vi "Periodic Tasks.vi"(11 "error out":errorcluster) -> ()   [LabVIEW 2013]
doc: "This VI runs in parallel to other tasks. It can contain as many user-defined periodic loops as you need. These can carry out PID or other sorts of timed response."
uses:
  <vilib>/Rock Robotics/SystemInterfaces/Utilities/FPGA_UtilitiesLED Source.ctl
  <vilib>/Rock Robotics/SystemInterfaces/Utilities/FPGA_UtilitiesLED State.ctl
  Robot Global Data.vi
  <vilib>/Rock Robotics/WPI/Joystick/WPI_JoystickGetSetRefNum.vi
  <vilib>/addons/control/pid/pid.llb/PID (DBL).vi
  <vilib>/addons/control/pid/NI_PID_pid.lvlib
  <vilib>/addons/Kinect/Skeleton Vertex Index.ctl
  <vilib>/addons/Kinect/SkeletonVertexTrackState.ctl
panel:
  out "x < y?":bool
  in  "Angle 2":i32=170
  in  "y 6":dbl=53.0
  in  "y 5":dbl=54.0
  in  "Drive PID":T1={"proportional gain (Kc)"=1.0, "integral time (Ti, min)"=0.01, "derivative time (Td, min)"=0.0} {"derivative time (Td, min)" format="%.3f"; "integral time (Ti, min)" format="%.3f"; "proportional gain (Kc)" format="%.3f"}
  in  "Joystick Multiplier":dbl=24.0
  in  "RateDivision":dbl=128.0
  out "Angle":dbl
  in  "Gyro PID":bool
  in  "PID gains 4":T1={"proportional gain (Kc)"=0.09999999999999999, "integral time (Ti, min)"=0.0, "derivative time (Td, min)"=0.002} {"derivative time (Td, min)" format="%.3f"; "integral time (Ti, min)" format="%.3f"; "proportional gain (Kc)" format="%.3f"}
  in  "SetFeeder":dbl=0.5
  in  "Encoder PID":bool
  in  "Reset Encoders":bool
  in  "y 4":i32=40
  in  "lower limit":dbl
  in  "y 3":i32=30
  in  "x":dbl=1.0
  in  "y 2":i32=2
  in  "y":i32=10
  in  "Gain (VoltsPerDegree/Second)":dbl=0.006999999999999999
  in  "Reset Gyro":bool
  in  "Encoder PID gains 2":T1={"proportional gain (Kc)"=0.30000000000000004, "integral time (Ti, min)"=0.0, "derivative time (Td, min)"=0.0}
  in  "Fly Speed 1":dbl(slide)=64.0 scale=0.0..100.0
  in  "Fly Speed 2":dbl(slide)=63.0 scale=0.0..100.0
  in  "Shooter Speed":T1={"proportional gain (Kc)"=0.13999999999999999, "integral time (Ti, min)"=0.0, "derivative time (Td, min)"=0.0} {"derivative time (Td, min)" format="%.3f"; "integral time (Ti, min)" format="%.3f"; "proportional gain (Kc)" format="%.3f"}
  in  "Fly 1":dbl
  in  "Fly 2":dbl
  out "Fly1 Rate":dbl
  out "Fly2 Rate":dbl
  in  "Reset Fly 2":bool
  in  "Reset Fly 1":bool
  out "Fly1":dbl
  out "Fly2":dbl
  in  "Encoder PID gains":T1={"proportional gain (Kc)"=0.30000000000000004, "integral time (Ti, min)"=0.0, "derivative time (Td, min)"=0.0}
  out "Drive Right feet":dbl
  out "Drive Left feet":dbl
  out "Drive Right":dbl
  out "Drive Left":dbl
  in  "PID gains 3":T1={"proportional gain (Kc)"=0.15, "integral time (Ti, min)"=0.0, "derivative time (Td, min)"=0.001} {"derivative time (Td, min)" format="%.3f"; "integral time (Ti, min)" format="%.3f"; "proportional gain (Kc)" format="%.3f"}
  # ".7 Front\n.5 Back"
  # "54/53 Front\n64/63 Back"
  # "-.72"
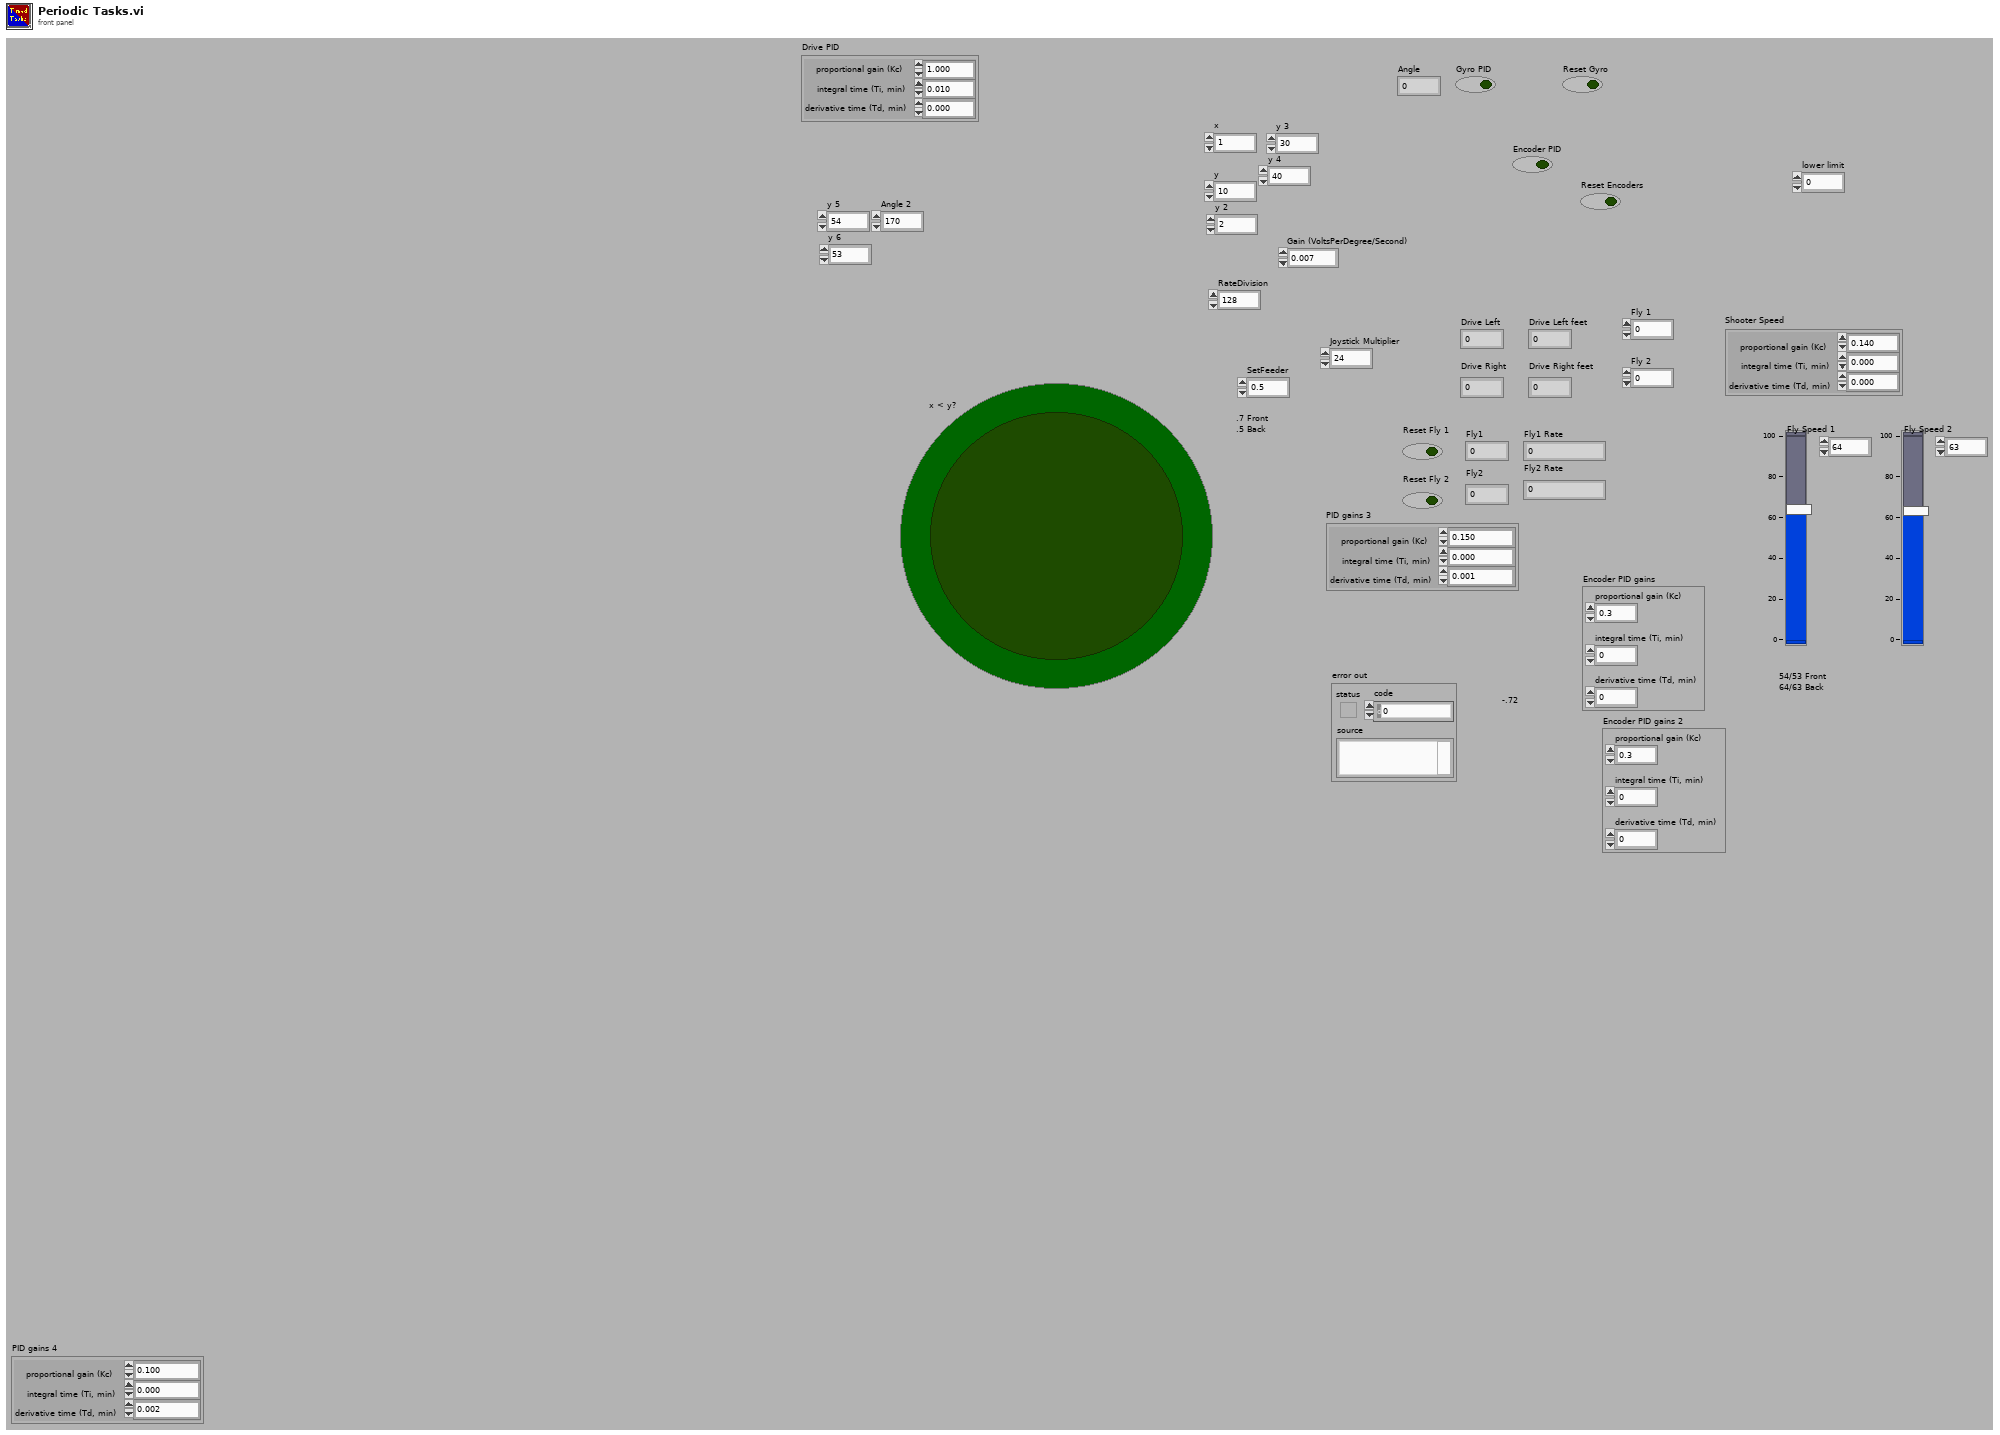
[diagram p1: front panel]
types:
  T1 = cluster{"proportional gain (Kc)":dbl, "integral time (Ti, min)":dbl, "derivative time (Td, min)":dbl}
  T2 = typedef "FPGA_UtilitiesLED State.ctl" = enum16{"Off", "On", "Toggle"}
  T3 = typedef "FPGA_UtilitiesLED Source.ctl" = enum16{"User LED", "FPGA LED"}
  T4 = typedef "WPI_MotorControlDeviceRef.ctl" = cluster{"DeviceStatus":errorcluster, "Type":enum16{"PWM", "CAN"}, "PWM":cluster{"Digital Module":T5, "PWM Channel":T6, "DeadBand":T7}, "CAN":cluster{"Device Number":u8, "Control Mode":T8, "Semaphore":T9, "Max Vout":dbl}, "Invert":bool, "TransformRef":T10, "InvTransformRef":T10}
  T5 = typedef "FPGA_TypedefDigitalModule.ctl" = enum16{"Digital Module 1", "Digital Module 2"}
  T6 = typedef "FPGA_DIOPWMChannel.ctl" = enum8{"PWM 1", "PWM 2", "PWM 3", "PWM 4", "PWM 5", "PWM 6", "PWM 7", "PWM 8", "PWM 9", "PWM 10", "Invalid"}
  T7 = typedef "WPI_PWMDeadband.ctl" = cluster{"Name":string, "maxPositivePwm":i32, "minPositivePwm":i32, "centerPwm":i32, "maxNegativePwm":i32, "minNegativePwm":i32, "angularRange":u16}
  T8 = typedef "WPI_CANJaguar_ControlMode.ctl" = enum8{"Percent VBus", "Current", "Speed", "Position", "Voltage"}
  T9 = typedef "Semaphore RefNum" = refnum<k1>
  T10 = typedef "WPI_PWMTransform_ConPane.ctl" = refnum<vi>
  T11 = typedef "WPI_EncoderDevRef.ctl" = cluster{"DevStatus":errorcluster, "EncoderIndex":T12, "CounterIndex":T13, "DistancePerCount":dbl, "Decoding Type":T14}
  T12 = typedef "FPGA_EncoderIdx.ctl" = enum8{"Enc 0", "Enc 1", "Enc 2", "Enc 3", "Invalid"}
  T13 = typedef "FPGA_CounterCtrSystemIndex.ctl" = enum8{"Ctr 0", "Ctr 1", "Ctr 2", "Ctr 3", "Ctr 4", "Ctr 5", "Ctr 6", "Ctr 7", "Invalid"}
  T14 = typedef "WPI_EncoderType.ctl" = enum16{"1x", "2x", "4x"}
  T15 = typedef "WPI_ServoDeviceRef.ctl" = cluster{"DeviceStatus":errorcluster, "Digital Module":T5, "PWM Channel":T6, "DeadBand":T7}
  T16 = typedef "WPI_JoystickDevRef.ctl" = cluster{"Device":T17}
  T17 = typedef "WPI_JoystickDeviceEnum.ctl" = enum16{"USB 1", "USB 2", "USB 3", "USB 4", "Kinect 1", "Kinect 2"}
  T18 = typedef "WPI_GyroDevRef.ctl" = cluster{"DevStatus":errorcluster, "Analog Module":T19, "Analog Channel":T20, "Offset":dbl, "Gain (VoltsPerDegree/Second)":dbl}
  T19 = typedef "FPGA_TypedefAnalogModule.ctl" = enum16{"Analog Module 1", "Analog Module 2"}
  T20 = typedef "FPGA_AIChannel.ctl" = enum8{"AI 1", "AI 2", "AI 3", "AI 4", "AI 5", "AI 6", "AI 7", "AI 8", "Invalid"}
  T21 = cluster{"axis 1 (x)":dbl, "axis 2 (y)":dbl, "axis 3 (throttle)":dbl, "axis 4":dbl, "axis 5":dbl, "axis 6":dbl}
  T22 = typedef "Skeleton Vertex Index.ctl" = i32
  T23 = typedef "SkeletonVertexTrackState.ctl" = enum32{"NotTracked", "Inferred", "Tracked"}
  T24 = cluster{"Target Info 2":cluster{"Center Position":cluster{"X":dbl, "Y":dbl}, "Distance (ft)":dbl, "Center":bool, "Angle":dbl}[]}
  T25 = cluster{"Center Position":cluster{"X":dbl, "Y":dbl}, "Distance (ft)":dbl, "Center":bool, "Angle":dbl}[]
  T26 = typedef "WPI_JoystickButtonState.ctl" = cluster{"Button 1":bool, "Button 2":bool, "Button 3":bool, "Button 4":bool, "Button 5":bool, "Button 6":bool, "Button 7":bool, "Button 8":bool, "Button 9":bool, "Button 10":bool, "Button 11":bool, "Button 12":bool}
  T27 = cluster{"Target Info 2[0]":cluster{"Center Position":cluster{"X":dbl, "Y":dbl}, "Distance (ft)":dbl, "Center":bool, "Angle":dbl}, "Target Info 2[1]":cluster{"Center Position":cluster{"X":dbl, "Y":dbl}, "Distance (ft)":dbl, "Center":bool, "Angle":dbl}, "Target Info 2[2]":cluster{"Center Position":cluster{"X":dbl, "Y":dbl}, "Distance (ft)":dbl, "Center":bool, "Angle":dbl}, "Target Info 2[3]":cluster{"Center Position":cluster{"X":dbl, "Y":dbl}, "Distance (ft)":dbl, "Center":bool, "Angle":dbl}, "Target Info 2[4]":cluster{"Center Position":cluster{"X":dbl, "Y":dbl}, "Distance (ft)":dbl, "Center":bool, "Angle":dbl}, "Target Info 2[5]":cluster{"Center Position":cluster{"X":dbl, "Y":dbl}, "Distance (ft)":dbl, "Center":bool, "Angle":dbl}, "Target Info 2[6]":cluster{"Center Position":cluster{"X":dbl, "Y":dbl}, "Distance (ft)":dbl, "Center":bool, "Angle":dbl}, "Target Info 2[7]":cluster{"Center Position":cluster{"X":dbl, "Y":dbl}, "Distance (ft)":dbl, "Center":bool, "Angle":dbl}, "Target Info 2[8]":cluster{"Center Position":cluster{"X":dbl, "Y":dbl}, "Distance (ft)":dbl, "Center":bool, "Angle":dbl}}
  T28 = cluster{"Center Position":cluster{"X":dbl, "Y":dbl}, "Distance (ft)":dbl, "Center":bool, "Angle":dbl}
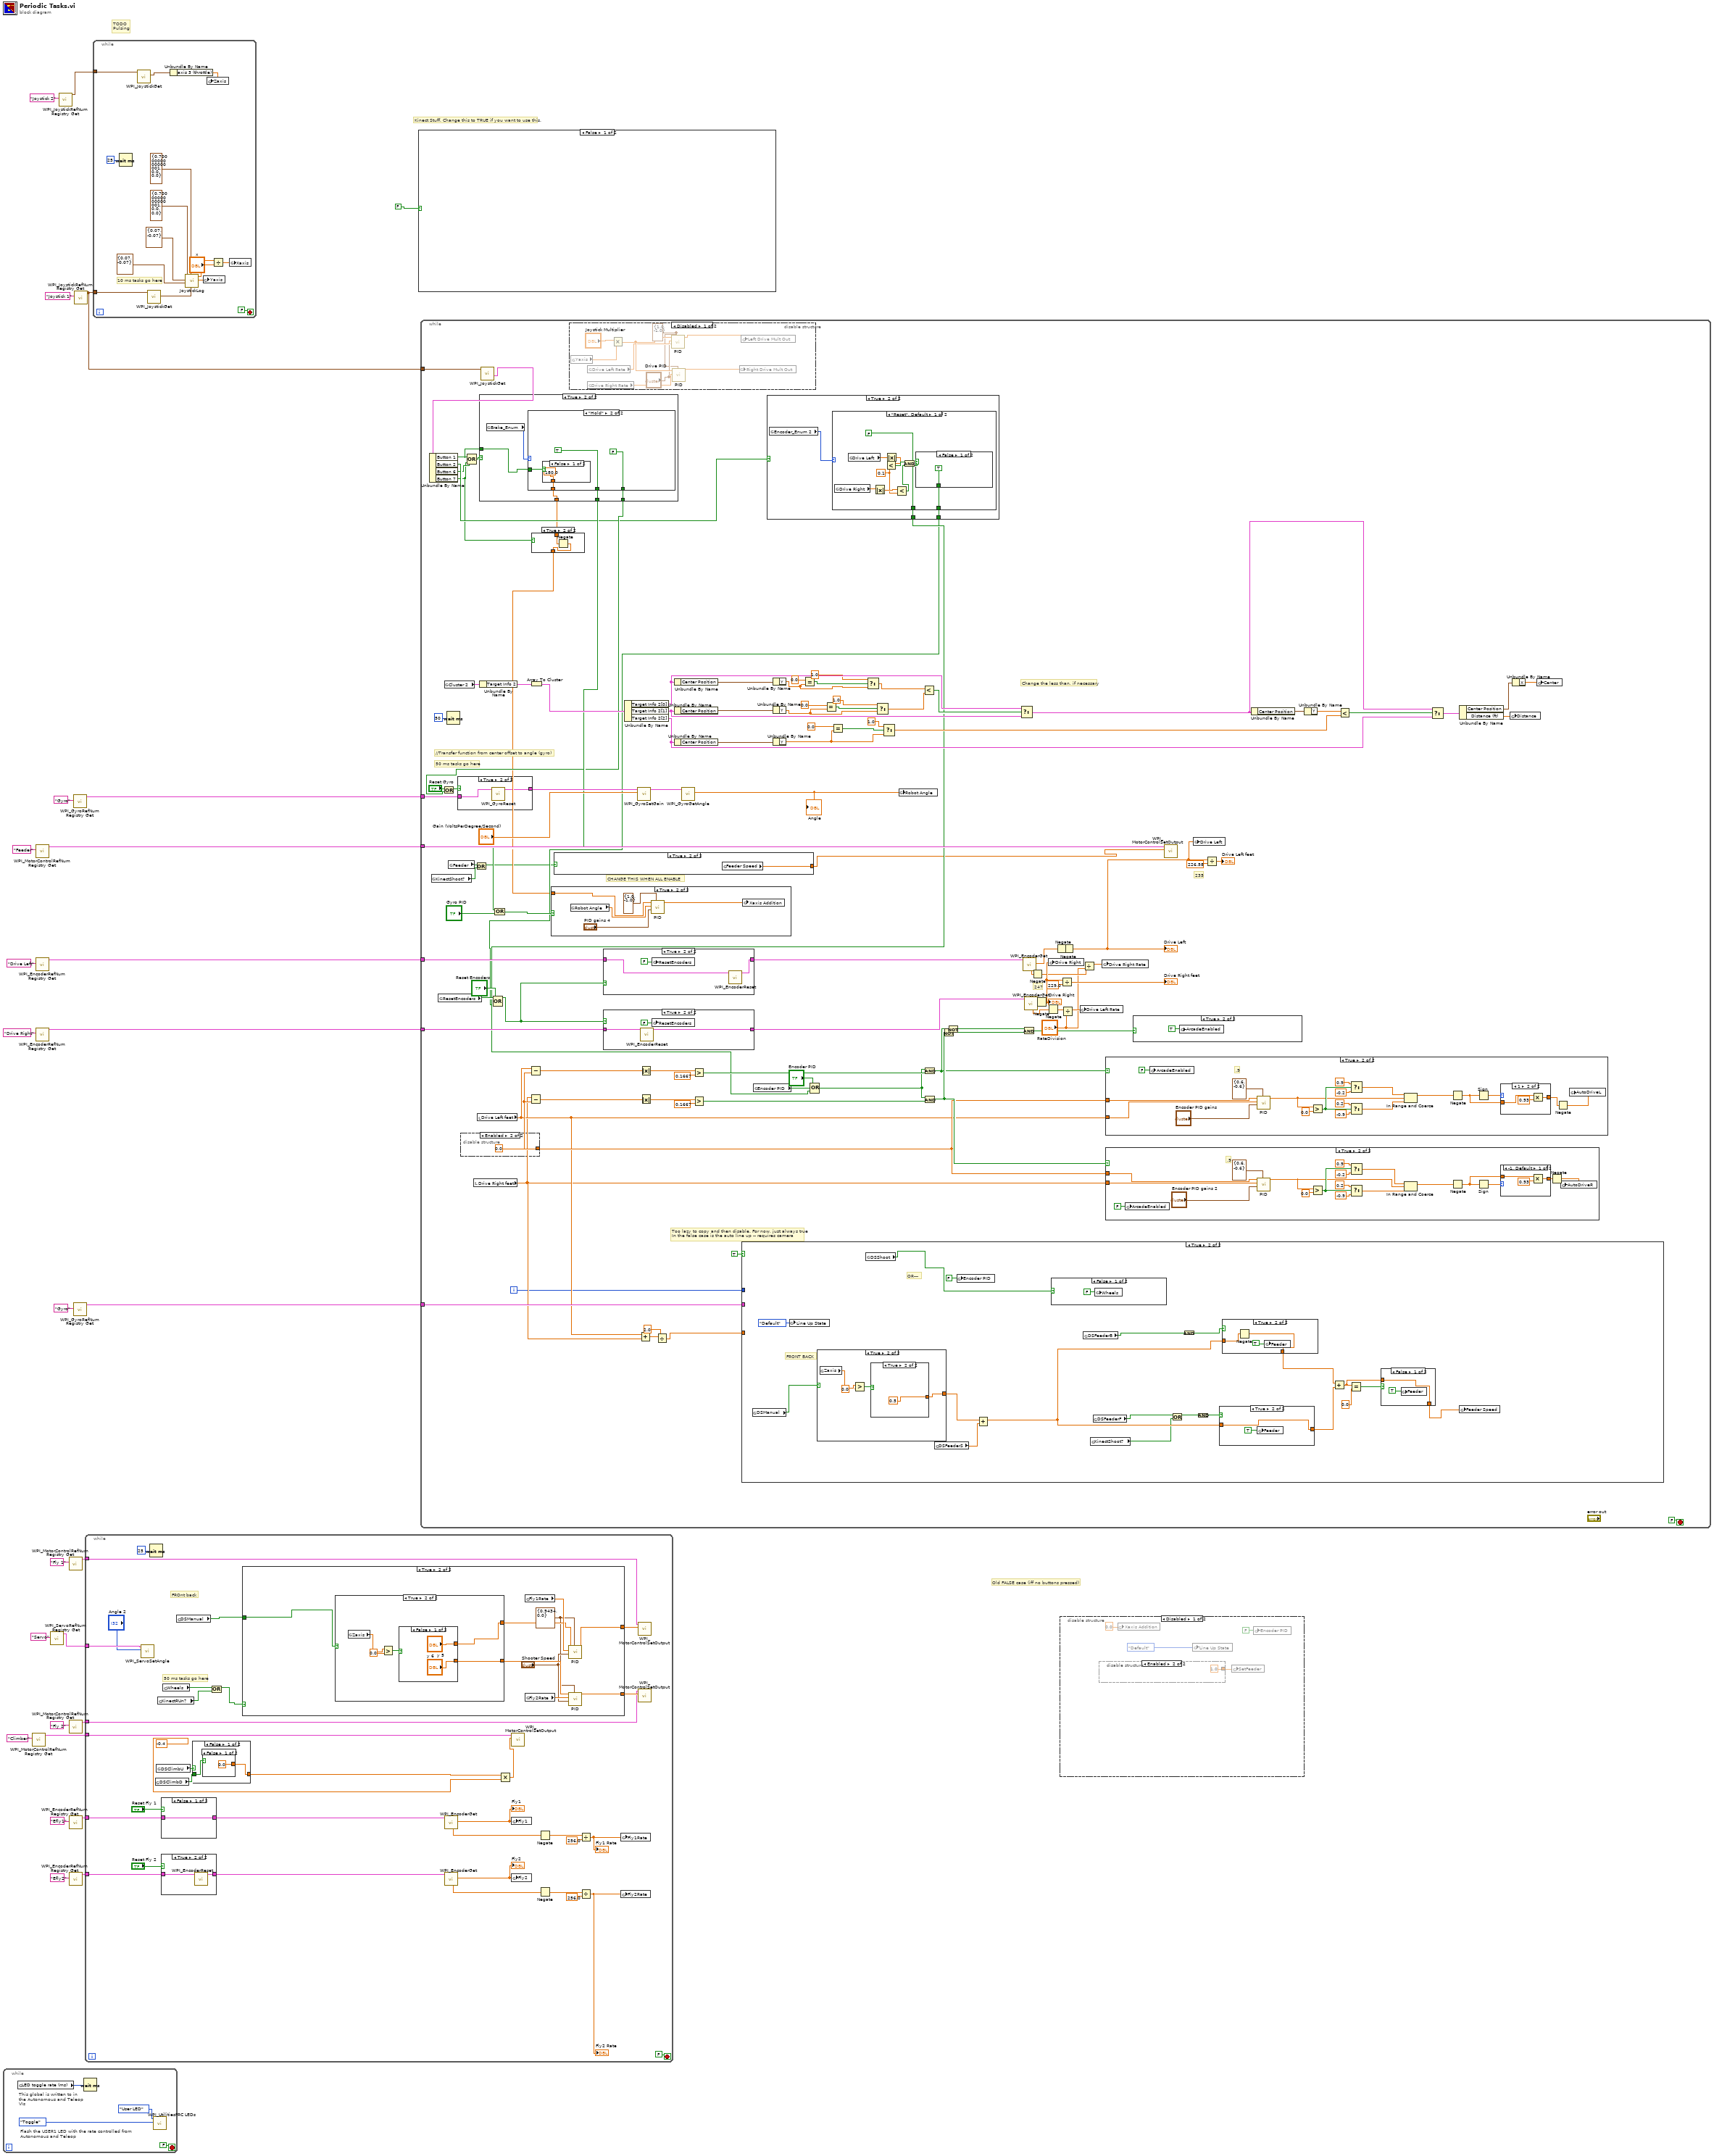
[diagram p0: block diagram]
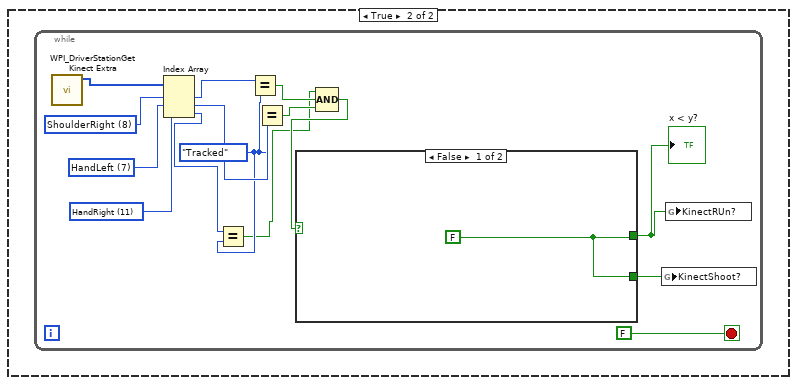
[diagram p2: hidden frame]
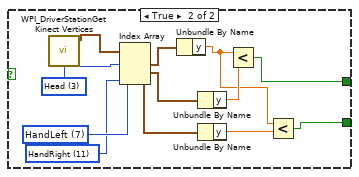
[diagram p3: hidden frame]
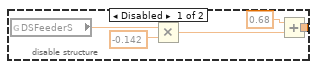
[diagram p4: hidden frame]
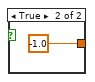
[diagram p6: hidden frame]
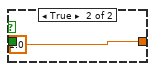
[diagram p7: hidden frame]
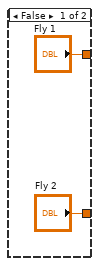
[diagram p8: hidden frame]
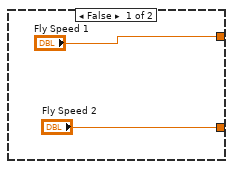
[diagram p9: hidden frame]
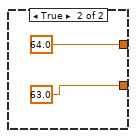
[diagram p10: hidden frame]
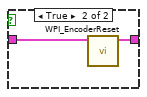
[diagram p11: hidden frame]
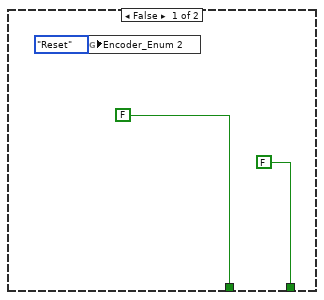
[diagram p14: hidden frame]
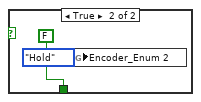
[diagram p15: hidden frame]
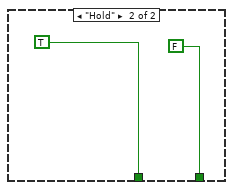
[diagram p16: hidden frame]
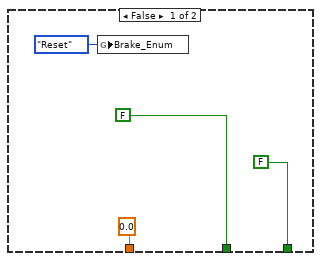
[diagram p18: hidden frame]
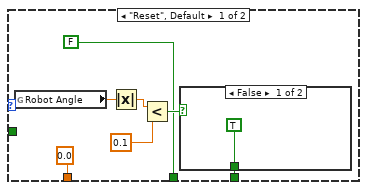
[diagram p19: hidden frame]
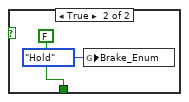
[diagram p20: hidden frame]
diagram:
  # "Kinect Stuff. Change this to TRUE if you want to use this."
  # "Old FALSE case (iff no buttons pressed)"
  # "TODO\nPulsing"
  n1 = while {
    stop <- FALSE stop-if-true
    # "This global is written to in the Autonomous and Teleop VIs"
    # "Flash the USER1 LED with the rate controlled from Autonomous and Teleop"
    n2 = global read "Robot Global Data.vi" "LED toggle rate (ms)"() -> (w28:u32)
    n3 = Wait (ms)(milliseconds to wait=w28) -> ()  [unwired: 1 out]
    n4 = call <vilib>:"WPI_UtilitiesFRC LEDs.vi"("State"=FPGA_UtilitiesLED_State."Toggle", "LED Type"=FPGA_UtilitiesLED_Source."User LED") -> ()  [unwired: 1 in, 9 out]
  }
  n5 = call <vilib>:"WPI_MotorControlRefNum Registry Get.vi"("refnum name"="Climber") -> ("MotorControlDevRef"=w11:T4)  [unwired: 9 in, 1 out]
  n6 = call <vilib>:"WPI_MotorControlRefNum Registry Get.vi"("refnum name"="Feeder") -> ("MotorControlDevRef"=w23:T4)  [unwired: 9 in, 1 out]
  n7 = call <vilib>:"WPI_EncoderRefNum Registry Get.vi"("refnum name"="Drive Left") -> ("EncoderDevRef"=w25:T11)  [unwired: 9 in, 1 out]
  n8 = call <vilib>:"WPI_EncoderRefNum Registry Get.vi"("refnum name"="Drive Right") -> ("EncoderDevRef"=w21:T11)  [unwired: 9 in, 1 out]
  n9 = call <vilib>:"WPI_ServoRefNum Registry Get.vi"("refnum name"="Servo") -> ("ServoDeviceRef"=w3:T15)  [unwired: 9 in, 1 out]
  n10 = call <vilib>:"WPI_JoystickRefNum Registry Get.vi"("refnum name"="Joystick 2") -> ("JoystickDevRef"=w4:T16)  [unwired: 1 in, 9 out]
  n11 = call <vilib>:"WPI_MotorControlRefNum Registry Get.vi"("refnum name"="Fly 1") -> ("MotorControlDevRef"=w14:T4)  [unwired: 9 in, 1 out]
  n12 = call <vilib>:"WPI_MotorControlRefNum Registry Get.vi"("refnum name"="Fly 2") -> ("MotorControlDevRef"=w13:T4)  [unwired: 9 in, 1 out]
  n13 = call <vilib>:"WPI_EncoderRefNum Registry Get.vi"("refnum name"="Efly1") -> ("EncoderDevRef"=w18:T11)  [unwired: 9 in, 1 out]
  n14 = call <vilib>:"WPI_EncoderRefNum Registry Get.vi"("refnum name"="Efly2") -> ("EncoderDevRef"=w17:T11)  [unwired: 9 in, 1 out]
  n15 = call <vilib>:"WPI_GyroRefNum Registry Get.vi"("refnum name"="Gyro") -> ("GyroDevRef"=w26:T18)  [unwired: 9 in, 1 out]
  n16 = call <vilib>:"WPI_GyroRefNum Registry Get.vi"("refnum name"="Gyro") -> ("GyroDevRef"=w24:T18)  [unwired: 9 in, 1 out]
  n17 = call <vilib>:"WPI_JoystickRefNum Registry Get.vi"("refnum name"="Joystick 1") -> ("JoystickDevRef"=w6:T16)  [unwired: 1 in, 9 out]
  n18 = while {
    tunnel: w18 -> [w52]
    tunnel: w17 -> [w54]
    tunnel: w14 -> [w47]
    tunnel: w13 -> [w46]
    tunnel: w11 -> [w42]
    tunnel: w3 -> [w35]
    stop <- FALSE stop-if-true
    # "FROnt back"
    # "50 ms tasks go here"
    n19 = call <vilib>:"WPI_ServoSetAngle.vi"("Angle"="Angle 2", "ServoDeviceRef"=w35) -> ()  [unwired: 8 in, 2 out]
    n20 = Wait (ms)(milliseconds to wait=u32 25) -> ()  [unwired: 1 out]
    n21 = global read "Robot Global Data.vi" "DSClimbD"() -> (w38:bool)
    n22 = global read "Robot Global Data.vi" "DSClimbU"() -> (w43:bool)
    n23 = global read "Robot Global Data.vi" "KinectRUn?"() -> (w32:bool)
    n24 = case shown="False" "Reset Fly 1" {
      tunnel: w52 -> [w93 w95]
      tunnel: [w93 w94] -> w51
      frame False {
      }
      frame True {
        n25 = call <vilib>:"WPI_EncoderReset.vi"("EncoderDevRef"=w95) -> ("EncoderDevRef"=w94:T11)  [unwired: 9 in, 1 out]
      }
    }
    n26 = case shown="True" "Reset Fly 2" {
      tunnel: w54 -> [w96 w97]
      tunnel: [w96 w98] -> w50
      frame False {
      }
      frame True {
        n27 = call <vilib>:"WPI_EncoderReset.vi"("EncoderDevRef"=w97) -> ("EncoderDevRef"=w98:T11)  [unwired: 9 in, 1 out]
      }
    }
    n28 = global read "Robot Global Data.vi" "Wheels"() -> (w37:bool)
    n29 = global read "Robot Global Data.vi" "DSManual"() -> (w36:bool)
    n30 = case shown="False" w43 {
      tunnel: [w67 1.0 ("y")] -> w40
      tunnel: w38 -> [w66 _]
      frame False {
        n31 = case shown="False" w66 {
          tunnel: [0.0 ("y") -1.0 ("y")] -> w67
          frame False {
          }
          frame True {
          }
        }
      }
      frame True {
      }
    }
    n32 = Or(x=w37, y=w32) -> (x .or. y?=w33:bool)
    n33 = case shown="True" w33 {
      tunnel: ["Fly 1" w75] -> w49
      tunnel: ["Fly 2" w74] -> w48
      tunnel: w36 -> [_ w73]
      frame False {
      }
      frame True {
        w76 = cluster{"output high":dbl, "output low":dbl} {"output high"=0.9434, "output low"=0.0} ("output range")
        n34 = case shown="True" w73 {
          tunnel: ["Fly Speed 1" w85] -> w80
          tunnel: ["Fly Speed 2" w84] -> w79
          frame False {
          }
          frame True {
            n35 = global read "Robot Global Data.vi" "Zaxis"() -> (w88:dbl)
            n36 = Greater?(x=w88, y=0.0) -> (0:w86:bool)
            n37 = case shown="False" w86 {
              tunnel: ["y 5" 64.0 ("y")] -> w85
              tunnel: ["y 6" 63.0 ("y")] -> w84
              frame False {
              }
              frame True {
              }
            }
          }
        }
        n38 = global read "Robot Global Data.vi" "Fly1Rate"() -> (w81:dbl)
        n39 = global read "Robot Global Data.vi" "Fly2Rate"() -> (w78:dbl)
        n40 = call-poly <vilib>:"PID.vi"("output range"=w76, "PID gains"="Shooter Speed", "process variable"=w81, "setpoint"=w80) -> ("output"=w75:dbl)  [unwired: 6 in, 1 out]
        n41 = call-poly <vilib>:"PID.vi"("output range"=w76, "PID gains"="Shooter Speed", "process variable"=w78, "setpoint"=w79) -> ("output"=w74:dbl)  [unwired: 6 in, 1 out]
      }
    }
    n42 = call <vilib>:"WPI_EncoderGet.vi"("EncoderDevRef"=w51) -> ("Distance"=w64:dbl, "Rate"=w55:dbl)  [unwired: 5 in, 4 out]
    "Fly1" <- w64
    n43 = call <vilib>:"WPI_EncoderGet.vi"("EncoderDevRef"=w50) -> ("Distance"=w63:dbl, "Rate"=w62:dbl)  [unwired: 5 in, 4 out]
    "Fly2" <- w63
    n44 = Multiply(x=w40, y=-0.4) -> (x*y=w41:dbl)
    n45 = call <vilib>:"WPI_MotorControlSetOutput.vi"("Output"=w41, "MotorControlDevRef"=w42) -> ()  [unwired: 7 in, 3 out]
    n46 = global write "Robot Global Data.vi" "Fly1"(w64) -> ()
    n47 = global write "Robot Global Data.vi" "Fly2"(w63) -> ()
    n48 = Negate(x=w55) -> (-x=w57:dbl)
    n49 = Negate(x=w62) -> (-x=w56:dbl)
    n50 = Divide(x=w57, y=256.0) -> (x/y=w59:dbl)
    "Fly1 Rate" <- w59
    n51 = Divide(x=w56, y=256.0) -> (x/y=w58:dbl)
    "Fly2 Rate" <- w58
    n52 = global write "Robot Global Data.vi" "Fly1Rate"(w59) -> ()
    n53 = global write "Robot Global Data.vi" "Fly2Rate"(w58) -> ()
    n54 = call <vilib>:"WPI_MotorControlSetOutput.vi"("Output"=w49, "MotorControlDevRef"=w47) -> ()  [unwired: 7 in, 3 out]
    n55 = call <vilib>:"WPI_MotorControlSetOutput.vi"("Output"=w48, "MotorControlDevRef"=w46) -> ()  [unwired: 7 in, 3 out]
  }
  n56 = while {
    tunnel: w6 -> [w111]
    tunnel: w4 -> [w101]
    stop <- FALSE stop-if-true
    # "10 ms tasks go here"
    n57 = Wait (ms)(milliseconds to wait=u32 25) -> ()  [unwired: 1 out]
    n58 = call <vilib>:"WPI_JoystickGet.vi"("JoystickDevRef"=w101) -> ("Axes"=w100:T21)  [unwired: 4 in, 2 out]
    n59 = call <vilib>:"WPI_JoystickGet.vi"("JoystickDevRef"=w111) -> ("Axes"=w112:T21)  [unwired: 4 in, 2 out]
    n60 = Unbundle By Name(w100) -> ("axis 3 (throttle)"=w99:dbl)
    n61 = call "JoystickLog.vi"("Axes"=w112, "PID y"=T1 {"proportional gain (Kc)"=0.7000000000000001, "integral time (Ti, min)"=0.0, "derivative time (Td, min)"=0.0}, "XMAXMIN"=cluster{"output high":dbl, "output low":dbl} {"output high"=0.07, "output low"=-0.07}, "YMAXMIN"=cluster{"output high":dbl, "output low":dbl} {"output high"=0.07, "output low"=-0.07}, "PID x"=T1 {"proportional gain (Kc)"=0.7000000000000001, "integral time (Ti, min)"=0.0, "derivative time (Td, min)"=0.0}) -> ("upper limit"=w104:dbl, "upper limit 2"=w105:dbl)  [unwired: 5 in]
    n62 = global write "Robot Global Data.vi" "Yaxis"(w104) -> ()
    n63 = global write "Robot Global Data.vi" "Zaxis"(w99) -> ()
    n64 = Divide(x=w105, y="x") -> (x/y=w103:dbl)
    n65 = global write "Robot Global Data.vi" "Xaxis"(w103) -> ()
  }
  n66 = case shown="False" FALSE {
    frame False {
    }
    frame True {
      n67 = while {
        stop <- FALSE stop-if-true
        w118 = T22 11 items=["HipCenter", "Spine", "ShoulderCenter", "Head", "ShoulderLeft", "ElbowLeft", "WristLeft", "HandLeft", "ShoulderRight", "ElbowRight", "WristRight", "HandRight", "HipLeft", "KneeLeft", "AnkleLeft", "FootLeft", "HipRight", "KneeRight", "AnkleRight", "FootRight"] ("Skeleton Joints")
        w116 = SkeletonVertexTrackState."Tracked" ("x")
        w125 = T22 7 items=["HipCenter", "Spine", "ShoulderCenter", "Head", "ShoulderLeft", "ElbowLeft", "WristLeft", "HandLeft", "ShoulderRight", "ElbowRight", "WristRight", "HandRight", "HipLeft", "KneeLeft", "AnkleLeft", "FootLeft", "HipRight", "KneeRight", "AnkleRight", "FootRight"] ("Skeleton Joints")
        w126 = T22 8 items=["HipCenter", "Spine", "ShoulderCenter", "Head", "ShoulderLeft", "ElbowLeft", "WristLeft", "HandLeft", "ShoulderRight", "ElbowRight", "WristRight", "HandRight", "HipLeft", "KneeLeft", "AnkleLeft", "FootLeft", "HipRight", "KneeRight", "AnkleRight", "FootRight"] ("Skeleton Joints")
        n68 = call <vilib>:"WPI_DriverStationGet Kinect Extra.vi"() -> ("Skeleton Tracking State"=w127:T23[])  [unwired: 7 in, 4 out]
        n69 = Index Array(array=w127, index #1=w126, index #2=w125, index #3=w118) -> (element #1=w124:T23, element #2=w123:T23, element #3=w117:T23)
        n70 = Equal?(x=w117, y=w116) -> (x = y?=w115:bool)
        n71 = Equal?(x=w124, y=w116) -> (x = y?=w122:bool)
        n72 = Equal?(x=w116, y=w123) -> (x = y?=w121:bool)
        n73 = Compound Arithmetic op=AND(w115, w122, w121) -> (w120:bool)
        n74 = case shown="False" w120 {
          tunnel: [w129 w135] -> w119
          tunnel: [w129 w130] -> w114
          frame False {
            w129 = FALSE
          }
          frame True {
            w134 = T22 11 items=["HipCenter", "Spine", "ShoulderCenter", "Head", "ShoulderLeft", "ElbowLeft", "WristLeft", "HandLeft", "ShoulderRight", "ElbowRight", "WristRight", "HandRight", "HipLeft", "KneeLeft", "AnkleLeft", "FootLeft", "HipRight", "KneeRight", "AnkleRight", "FootRight"] ("Skeleton Joints")
            w139 = T22 7 items=["HipCenter", "Spine", "ShoulderCenter", "Head", "ShoulderLeft", "ElbowLeft", "WristLeft", "HandLeft", "ShoulderRight", "ElbowRight", "WristRight", "HandRight", "HipLeft", "KneeLeft", "AnkleLeft", "FootLeft", "HipRight", "KneeRight", "AnkleRight", "FootRight"] ("Skeleton Joints")
            w140 = T22 3 items=["HipCenter", "Spine", "ShoulderCenter", "Head", "ShoulderLeft", "ElbowLeft", "WristLeft", "HandLeft", "ShoulderRight", "ElbowRight", "WristRight", "HandRight", "HipLeft", "KneeLeft", "AnkleLeft", "FootLeft", "HipRight", "KneeRight", "AnkleRight", "FootRight"] ("Skeleton Joints")
            n75 = call <vilib>:"WPI_DriverStationGet Kinect Vertices.vi"() -> ("Skeleton Vertices"=w141:cluster{"x":sgl, "y":sgl, "z":sgl}[])  [unwired: 10 in, 1 out]
            n76 = Index Array(array=w141, index #1=w140, index #2=w139, index #3=w134) -> (element #1=w138:cluster{"x":sgl, "y":sgl, "z":sgl}, element #2=w137:cluster{"x":sgl, "y":sgl, "z":sgl}, element #3=w133:cluster{"x":sgl, "y":sgl, "z":sgl})
            n77 = Unbundle By Name(w138) -> ("y"=w132:sgl)
            n78 = Unbundle By Name(w137) -> ("y"=w136:sgl)
            n79 = Unbundle By Name(w133) -> ("y"=w131:sgl)
            n80 = Less?(x=w132, y=w136) -> (x < y?=w135:bool)
            n81 = Less?(x=w132, y=w131) -> (x < y?=w130:bool)
          }
        }
        "x < y?" <- w119
        n82 = global write "Robot Global Data.vi" "KinectShoot?"(w114) -> ()
        n83 = global write "Robot Global Data.vi" "KinectRUn?"(w119) -> ()
      }
    }
  }
  n84 = while {
    tunnel: w26 -> [w248]
    tunnel: w25 -> [w245]
    tunnel: w24 -> [w247]
    tunnel: w23 -> [w249]
    tunnel: w21 -> [w246]
    tunnel: w6 -> [w167]
    i -> [w169]
    stop <- FALSE stop-if-true
    # "Too lazy to copy and then disable. For now, just always true\nIn the false case is the auto line up -- requires camera"
    # "247"
    # "235"
    # "50 ms tasks go here"
    # "//Transfer function from center offset to angle (gyro)"
    # "Change the less than, if necessary"
    # "CHANGE THIS WHEN ALL ENABLE"
    n85 = global read "Robot Global Data.vi" "KinectShoot?"() -> (w142:bool)
    n86 = global read "Robot Global Data.vi" "ResetEncoders"() -> (w174:bool)
    n87 = global read "Robot Global Data.vi" "Cluster 2"() -> (w239:T24)
    n88 = Wait (ms)(milliseconds to wait=u32 50) -> ()  [unwired: 1 out]
    n89 = global read "Robot Global Data.vi" "Feeder"() -> (w221:bool)
    n90 = disable-structure shown="Enabled" {
      disable-tunnel: [w316 0.0 ("EncoderDistance")] -> w209
      frame Disabled {
        n91 = global read "Robot Global Data.vi" "EncoderDistance"() -> (w316:dbl)
      }
      frame Enabled {
      }
    }
    n92 = local read "Drive Right feet"() -> (w178:dbl)
    n93 = Or(x=w221, y=w142) -> (x .or. y?=w143:bool)
    n94 = local read "Drive Left feet"() -> (w179:dbl)
    n95 = Unbundle By Name(w239) -> ("Target Info 2"=w240:T25)
    n96 = call <vilib>:"WPI_JoystickGet.vi"("JoystickDevRef"=w167) -> ("Buttons"=w166:T26)  [unwired: 4 in, 2 out]
    n97 = Unbundle By Name(w166) -> ("Button 1"=w149:bool, "Button 2"=w154:bool, "Button 6"=w150:bool, "Button 7"=w145:bool)
    n98 = Compound Arithmetic op=OR(w149, w150, w145) -> (w151:bool)
    n99 = case shown="True" w151 {
      tunnel: [FALSE w292] -> w164
      tunnel: [FALSE w291] -> w162
      tunnel: [0.0 ("setpoint") w289] -> w146
      tunnel: w149 -> [_ w290]
      frame False {
        n100 = global write "Robot Global Data.vi" "Brake_Enum"(enum16{"Reset", "Hold"}."Reset" ("Brake_Enum")) -> ()
      }
      frame True {
        n101 = global read "Robot Global Data.vi" "Brake_Enum"() -> (w293:enum16{"Reset", "Hold"})
        n102 = case shown="\"Hold\"" w293 {
          tunnel: [FALSE TRUE] -> w292
          tunnel: [w295 FALSE] -> w291
          tunnel: w290 -> [_ w305]
          tunnel: [0.0 ("setpoint") w304] -> w289
          frame "Reset", Default {
            n103 = global read "Robot Global Data.vi" "Robot Angle"() -> (w299:dbl)
            n104 = Absolute Value(x=w299) -> (abs(x)=w297:dbl)
            n105 = Less?(x=w297, y=0.1) -> (x < y?=w300:bool)
            n106 = case shown="False" w300 {
              tunnel: [TRUE FALSE] -> w295
              frame False {
              }
              frame True {
                n107 = global write "Robot Global Data.vi" "Brake_Enum"(enum16{"Reset", "Hold"}."Hold" ("Brake_Enum")) -> ()
              }
            }
          }
          frame "Hold" {
            n108 = case shown="False" w305 {
              tunnel: [180.0 ("setpoint") 0.0 ("setpoint")] -> w304
              frame False {
              }
              frame True {
              }
            }
          }
        }
      }
    }
    n109 = Or(x="Reset Gyro", y=w162) -> (x .or. y?=w163:bool)
    n110 = case shown="True" w163 {
      tunnel: w248 -> [w381 w383]
      tunnel: [w381 w382] -> w224
      frame False {
      }
      frame True {
        n111 = call <vilib>:"WPI_GyroReset.vi"("GyroDevRef"=w383) -> ("GyroDevRef"=w382:T18)  [unwired: 9 in, 1 out]
      }
    }
    n112 = Compound Arithmetic op=OR(w164, "Gyro PID") -> (w165:bool)
    n113 = Subtract(x=w179, y=w209) -> (x-y=w217:dbl)
    n114 = Subtract(x=w178, y=w209) -> (x-y=w216:dbl)
    n115 = Array To Cluster(array=w240) -> (cluster=w241:T27)
    n116 = case shown="True" w145 {
      tunnel: [w252 w253] -> w147
      tunnel: w146 -> [w252 w254]
      frame False {
      }
      frame True {
        n117 = Negate(x=w254) -> (-x=w253:dbl)
      }
    }
    n118 = case shown="True" w165 {
      tunnel: w147 -> [_ w311]
      frame False {
        n119 = global write "Robot Global Data.vi" "Xaxis Addition"(0.0 ("Xaxis Addition")) -> ()
      }
      frame True {
        n120 = global read "Robot Global Data.vi" "Robot Angle"() -> (w315:dbl)
        n121 = call-poly <vilib>:"PID.vi"("output range"=cluster{"output high":dbl, "output low":dbl} {"output high"=1.0, "output low"=-1.0}, "PID gains"="PID gains 4", "process variable"=w315, "setpoint"=w311) -> ("output"=w314:dbl)  [unwired: 6 in, 1 out]
        n122 = global write "Robot Global Data.vi" "Xaxis Addition"(w314) -> ()
      }
    }
    n123 = case shown="True" w143 {
      tunnel: [0.0 ("Feeder Addition") w503] -> w144
      frame False {
      }
      frame True {
        n124 = global read "Robot Global Data.vi" "Feeder Speed"() -> (w503:dbl)
      }
    }
    n125 = disable-structure shown="Disabled" {
      frame Disabled {
        w276 = cluster{"output high":dbl, "output low":dbl} {"output high"=1.0, "output low"=-1.0} ("output range")
        n126 = global read "Robot Global Data.vi" "Yaxis"() -> (w284:dbl)
        n127 = global read "Robot Global Data.vi" "Drive Right Rate"() -> (w281:dbl)
        n128 = global read "Robot Global Data.vi" "Drive Left Rate"() -> (w280:dbl)
        n129 = Multiply(x="Joystick Multiplier", y=w284) -> (x*y=w282:dbl)
        n130 = call-poly <vilib>:"PID.vi"("output range"=w276, "PID gains"="Drive PID", "process variable"=w280, "setpoint"=w282) -> ("output"=w278:dbl)  [unwired: 6 in, 1 out]
        n131 = call-poly <vilib>:"PID.vi"("output range"=w276, "PID gains"="Drive PID", "process variable"=w281, "setpoint"=w282) -> ("output"=w277:dbl)  [unwired: 6 in, 1 out]
        n132 = global write "Robot Global Data.vi" "Right Drive Mult Out"(w277) -> ()
        n133 = global write "Robot Global Data.vi" "Left Drive Mult Out"(w278) -> ()
      }
      frame Enabled {
      }
    }
    n134 = Unbundle By Name(w241) -> ("Target Info 2[0]"=w234:T28, "Target Info 2[1]"=w233:T28, "Target Info 2[2]"=w231:T28)
    n135 = call <vilib>:"WPI_GyroSetGain.vi"("Gain (VoltsPerDegree/Second)"="Gain (VoltsPerDegree/Second)", "GyroDevRef"=w224) -> ("GyroDevRef"=w223:T18)  [unwired: 8 in, 1 out]
    n136 = Add(x=w179, y=w178) -> (x+y=w177:dbl)
    n137 = Absolute Value(x=w217) -> (abs(x)=w220:dbl)
    n138 = Absolute Value(x=w216) -> (abs(x)=w213:dbl)
    n139 = Divide(x=w177, y=2.0) -> (x/y=w175:dbl)
    n140 = Unbundle By Name(w234) -> ("Center Position"=w238:cluster{"X":dbl, "Y":dbl})
    n141 = Unbundle By Name(w233) -> ("Center Position"=w237:cluster{"X":dbl, "Y":dbl})
    n142 = Unbundle By Name(w231) -> ("Center Position"=w236:cluster{"X":dbl, "Y":dbl})
    n143 = call <vilib>:"WPI_GyroGetAngle.vi"("GyroDevRef"=w223) -> ("Angle"=w225:dbl)  [unwired: 7 in, 3 out]
    "Angle" <- w225
    n144 = Greater?(x=w220, y=0.1667) -> (0:w219:bool)
    n145 = Greater?(x=w213, y=0.1667) -> (0:w214:bool)
    n146 = case shown="True" TRUE {
      tunnel: w247 -> [w387 _]
      tunnel: w169 -> [w386 _]
      tunnel: w175 -> [w384 _]
      frame False {
        n147 = global read "Robot Global Data.vi" "DSShoot"() -> (w385:bool)
        n148 = case shown="True" w385 {
          tunnel: w387 -> [_ w396]
          tunnel: w386 -> [_ w395]
          tunnel: w384 -> [_ w393]
          frame False {
            n149 = global write "Robot Global Data.vi" "Xaxis Addition"(0.0 ("Xaxis Addition")) -> ()
            n150 = global write "Robot Global Data.vi" "Feeder"(FALSE ("Feeder")) -> ()
            n151 = global write "Robot Global Data.vi" "Wheels"(FALSE ("Wheels")) -> ()
            n152 = global write "Robot Global Data.vi" "Line Up State"(enum16{"Default", "Gyro"}."Default" ("Line Up State")) -> ()
            n153 = global write "Robot Global Data.vi" "Encoder PID"(FALSE ("Encoder PID")) -> ()
          }
          frame True {
            n154 = global write "Robot Global Data.vi" "Wheels"(TRUE ("Wheels")) -> ()
            n155 = global read "Robot Global Data.vi" "Line Up State"() -> (w397:enum16{"Default", "Gyro", "Distance", "Shoot"})
            n156 = case shown="\"Shoot\"" w397 {
              tunnel: w396 -> [w407 _ _ _]
              tunnel: w395 -> [w400 w413 w438 w449]
              tunnel: w393 -> [_ _ w437 _]
              frame "Default", Default {
                n157 = global write "Robot Global Data.vi" "Iterator"(w400) -> ()
                n158 = global read "Robot Global Data.vi" "Center"() -> (w402:dbl)
                n159 = call <vilib>:"WPI_GyroReset.vi"("GyroDevRef"=w407) -> ()  [unwired: 9 in, 2 out]
                n160 = global write "Robot Global Data.vi" "ResetEncoders"(TRUE ("ResetEncoders")) -> ()
                n161 = Add(x=w402, y=0.1875 ("f")) -> (x+y=w403:dbl)
                n162 = global write "Robot Global Data.vi" "Encoder PID"(FALSE ("Encoder PID")) -> ()
                n163 = Multiply(x=w403, y=33.5) -> (x*y=w405:dbl)
                n164 = global write "Robot Global Data.vi" "Center Offset"(w405) -> ()
                n165 = Not Equal?(x=w405, y=0.0) -> (x != y?=w406:bool)
                n166 = case shown="False" w406 {
                  frame False {
                    n167 = global write "Robot Global Data.vi" "Line Up State"(enum16{"Default", "Gyro", "Distance", "Shoot"}."Distance" ("Line Up State")) -> ()
                  }
                  frame True {
                    n168 = global write "Robot Global Data.vi" "ResetEncoders"(TRUE ("ResetEncoders")) -> ()
                    n169 = global write "Robot Global Data.vi" "Line Up State"(enum16{"Default", "Gyro", "Distance", "Shoot"}."Distance" ("Line Up State")) -> ()
                  }
                }
              }
              frame "Gyro" {
                n170 = global read "Robot Global Data.vi" "Iterator"() -> (w417:i32)
                n171 = global read "Robot Global Data.vi" "Distance"() -> (w412:dbl)
                n172 = global read "Robot Global Data.vi" "Center Offset"() -> (w422:dbl)
                n173 = global read "Robot Global Data.vi" "Robot Angle"() -> (w421:dbl)
                n174 = Subtract(x=w413, y=w417) -> (x-y=w415:i32)
                n175 = global write "Robot Global Data.vi" "RobotDistance"(w412) -> ()
                n176 = Less?(x=w415, y="y 3") -> (x < y?=w414:bool)
                n177 = call-poly <vilib>:"PID.vi"("output range"=cluster{"output high":dbl, "output low":dbl} {"output high"=0.9, "output low"=-0.9}, "PID gains"="PID gains 3", "process variable"=w421, "setpoint"=w422) -> ("output"=w420:dbl)  [unwired: 6 in, 1 out]
                n178 = case shown="False" w414 {
                  tunnel: w413 -> [w425 _]
                  frame False {
                    n179 = global write "Robot Global Data.vi" "Iterator"(w425) -> ()
                    n180 = global write "Robot Global Data.vi" "ResetEncoders"(TRUE ("ResetEncoders")) -> ()
                    n181 = global write "Robot Global Data.vi" "Line Up State"(enum16{"Default", "Gyro", "Distance", "Shoot"}."Shoot" ("Line Up State")) -> ()
                  }
                  frame True {
                  }
                }
                n182 = global write "Robot Global Data.vi" "Xaxis Addition"(w420) -> ()
              }
              frame "Distance" {
                n183 = global read "Robot Global Data.vi" "Iterator"() -> (w434:i32)
                n184 = global write "Robot Global Data.vi" "Xaxis Addition"(0.0 ("Xaxis Addition")) -> ()
                n185 = Subtract(x=w438, y=w434) -> (x-y=w433:i32)
                n186 = global write "Robot Global Data.vi" "ResetEncoders"(FALSE ("ResetEncoders")) -> ()
                n187 = Greater?(x=w433, y="y 4") -> (0:w430:bool)
                n188 = In Range and Coerce(upper limit=2.0, x=w437, lower limit="lower limit") -> (In Range?=w427:bool)  [unwired: 1 out]
                n189 = Not(x=w427) -> (.not. x?=w426:bool)
                n190 = Or(x=w430, y=w426) -> (x .or. y?=w431:bool)
                n191 = case shown="True" w431 {
                  tunnel: w438 -> [_ w442]
                  frame False {
                    n192 = global write "Robot Global Data.vi" "Encoder PID"(TRUE ("Encoder PID")) -> ()
                    n193 = global write "Robot Global Data.vi" "EncoderDistance"(-5.65 ("y")) -> ()
                  }
                  frame True {
                    n194 = global write "Robot Global Data.vi" "Iterator"(w442) -> ()
                    n195 = global write "Robot Global Data.vi" "Encoder PID"(FALSE ("Encoder PID")) -> ()
                    n196 = global write "Robot Global Data.vi" "Line Up State"(enum16{"Default", "Gyro", "Distance", "Shoot"}."Shoot" ("Line Up State")) -> ()
                    n197 = global write "Robot Global Data.vi" "ResetEncoders"(TRUE ("ResetEncoders")) -> ()
                  }
                }
              }
              frame "Shoot" {
                # "OMG IT DID"
                n198 = Quotient & Remainder(x=w449, y="y") -> (floor(x/y)=w447:i32)  [unwired: 1 out]
                n199 = global write "Robot Global Data.vi" "Encoder PID"(FALSE ("Encoder PID")) -> ()
                n200 = Quotient & Remainder(x=w447, y="y 2") -> (x-y*floor(x/y)=w445:i32)  [unwired: 1 out]
                n201 = case shown="1" w445 {
                  frame 0, Default {
                    n202 = global write "Robot Global Data.vi" "Feeder"(FALSE ("Feeder")) -> ()
                  }
                  frame 1 {
                    n203 = global write "Robot Global Data.vi" "Feeder"(TRUE ("Feeder")) -> ()
                  }
                }
                n204 = disable-structure shown="Enabled" {
                  disable-tunnel: [w453 0.0 ("Feeder Speed")] -> w450
                  frame Disabled {
                    n205 = global read "Robot Global Data.vi" "Distance"() -> (w452:dbl)
                    n206 = Multiply(x=w452, y=-0.0650903132757) -> (x*y=w455:dbl)
                    n207 = Add(x=w455, y=1.6133553564946) -> (x+y=w453:dbl)
                  }
                  frame Enabled {
                  }
                }
                n208 = global write "Robot Global Data.vi" "Feeder Speed"(w450) -> ()
              }
            }
          }
        }
      }
      frame True {
        # "FRONT BACK"
        # "OR---"
        n209 = global read "Robot Global Data.vi" "DSManual"() -> (w462:bool)
        n210 = global write "Robot Global Data.vi" "Line Up State"(enum16{"Default", "Gyro", "Distance", "Shoot"}."Default" ("Line Up State")) -> ()
        n211 = case shown="True" w462 {
          tunnel: [w479 w483] -> w465
          frame False {
            n212 = disable-structure shown="Enabled" {
              disable-tunnel: [w480 w481] -> w479
              frame Disabled {
                n213 = global read "Robot Global Data.vi" "SetFeeder"() -> (w480:dbl)
              }
              frame Enabled {
                n214 = Absolute Value(x="SetFeeder") -> (abs(x)=w481:dbl)
              }
            }
          }
          frame True {
            n215 = global read "Robot Global Data.vi" "Zaxis"() -> (w486:dbl)
            n216 = Greater?(x=w486, y=0.0) -> (0:w484:bool)
            n217 = case shown="True" w484 {
              tunnel: [0.7 ("y") 0.5 ("y")] -> w483
              frame False {
              }
              frame True {
              }
            }
          }
        }
        n218 = global read "Robot Global Data.vi" "DSShoot"() -> (w476:bool)
        n219 = global read "Robot Global Data.vi" "DSFeederS"() -> (w463:dbl)
        n220 = global write "Robot Global Data.vi" "Encoder PID"(FALSE ("Encoder PID")) -> ()
        n221 = Add(x=w465, y=w463) -> (x+y=w464:dbl)
        n222 = case shown="False" w476 {
          frame False {
            n223 = global write "Robot Global Data.vi" "Wheels"(FALSE ("Wheels")) -> ()
          }
          frame True {
            n224 = global write "Robot Global Data.vi" "Wheels"(TRUE ("Wheels")) -> ()
          }
        }
        n225 = global read "Robot Global Data.vi" "DSFeederB"() -> (w478:bool)
        n226 = global read "Robot Global Data.vi" "KinectShoot?"() -> (w460:bool)
        n227 = global read "Robot Global Data.vi" "DSFeederF"() -> (w477:bool)
        n228 = Or(x=w477, y=w460) -> (x .or. y?=w461:bool)
        n229 = Compound Arithmetic op=AND(w478) -> (w473:bool)
        n230 = Compound Arithmetic op=AND(w461) -> (w472:bool)
        n231 = case shown="True" w472 {
          tunnel: [0.0 ("SetFeeder") w498] -> w470
          tunnel: w464 -> [_ w498]
          frame False {
          }
          frame True {
            n232 = global write "Robot Global Data.vi" "Feeder"(TRUE ("Feeder")) -> ()
          }
        }
        n233 = case shown="True" w473 {
          tunnel: [0.0 ("SetFeeder") w494] -> w471
          tunnel: w464 -> [_ w495]
          frame False {
          }
          frame True {
            n234 = Negate(x=w495) -> (-x=w494:dbl)
            n235 = global write "Robot Global Data.vi" "Feeder"(TRUE ("Feeder")) -> ()
          }
        }
        n236 = Add(x=w471, y=w470) -> (x+y=w466:dbl)
        n237 = Equal?(x=w466, y=0.0) -> (x = y?=w469:bool)
        n238 = case shown="False" w469 {
          tunnel: [w489 w492] -> w467
          tunnel: w466 -> [w489 w492]
          frame False {
            n239 = global write "Robot Global Data.vi" "Feeder"(TRUE ("Feeder")) -> ()
          }
          frame True {
            n240 = global write "Robot Global Data.vi" "Feeder"(FALSE ("Feeder")) -> ()
          }
        }
        n241 = global write "Robot Global Data.vi" "Feeder Speed"(w467) -> ()
      }
    }
    n242 = global read "Robot Global Data.vi" "Encoder PID"() -> (w208:bool)
    n243 = case shown="True" w154 {
      tunnel: [FALSE w259] -> w153
      tunnel: [FALSE w258] -> w152
      frame False {
        n244 = global write "Robot Global Data.vi" "Encoder_Enum 2"(enum16{"Reset", "Hold"}."Reset" ("Brake_Enum")) -> ()
      }
      frame True {
        n245 = global read "Robot Global Data.vi" "Encoder_Enum 2"() -> (w260:enum16{"Reset", "Hold"})
        n246 = case shown="\"Reset\", Default" w260 {
          tunnel: [FALSE TRUE] -> w259
          tunnel: [w266 FALSE] -> w258
          frame "Reset", Default {
            w264 = 0.1 ("y")
            n247 = global read "Robot Global Data.vi" "Drive Right"() -> (w261:dbl)
            n248 = global read "Robot Global Data.vi" "Drive Left"() -> (w269:dbl)
            n249 = Absolute Value(x=w261) -> (abs(x)=w265:dbl)
            n250 = Absolute Value(x=w269) -> (abs(x)=w268:dbl)
            n251 = Less?(x=w268, y=w264) -> (x < y?=w270:bool)
            n252 = Less?(x=w265, y=w264) -> (x < y?=w262:bool)
            n253 = And(x=w270, y=w262) -> (x .and. y?=w263:bool)
            n254 = case shown="False" w263 {
              tunnel: [TRUE FALSE] -> w266
              frame False {
              }
              frame True {
                n255 = global write "Robot Global Data.vi" "Encoder_Enum 2"(enum16{"Reset", "Hold"}."Hold" ("Brake_Enum")) -> ()
              }
            }
          }
          frame "Hold" {
          }
        }
      }
    }
    n256 = Compound Arithmetic op=OR(w174, "Reset Encoders", w152) -> (w173:bool)
    n257 = case shown="True" w173 {
      tunnel: [w318 w321] -> w207
      tunnel: w245 -> [w318 w320]
      frame False {
      }
      frame True {
        n258 = global write "Robot Global Data.vi" "ResetEncoders"(FALSE ("ResetEncoders")) -> ()
        n259 = call <vilib>:"WPI_EncoderReset.vi"("EncoderDevRef"=w320) -> ("EncoderDevRef"=w321:T11)  [unwired: 9 in, 1 out]
      }
    }
    n260 = case shown="True" w173 {
      tunnel: w246 -> [w322 w325]
      tunnel: [w322 w324] -> w206
      frame False {
      }
      frame True {
        n261 = call <vilib>:"WPI_EncoderReset.vi"("EncoderDevRef"=w325) -> ("EncoderDevRef"=w324:T11)  [unwired: 9 in, 1 out]
        n262 = global write "Robot Global Data.vi" "ResetEncoders"(FALSE ("ResetEncoders")) -> ()
      }
    }
    n263 = Unbundle By Name(w238) -> ("Y"=w193:dbl)
    n264 = Unbundle By Name(w237) -> ("Y"=w190:dbl)
    n265 = Unbundle By Name(w236) -> ("Y"=w185:dbl)
    n266 = Equal?(x=0.0, y=w193) -> (x = y?=w196:bool)
    n267 = Compound Arithmetic op=OR("Encoder PID", w208, w153) -> (w171:bool)
    n268 = Equal?(x=0.0, y=w190) -> (x = y?=w192:bool)
    n269 = Equal?(x=0.0, y=w185) -> (x = y?=w187:bool)
    n270 = Select(t=1.0, s=w196, f=w193) -> (s? t:f=w194:dbl)
    n271 = Select(t=1.0, s=w192, f=w190) -> (s? t:f=w189:dbl)
    n272 = Select(t=1.0, s=w187, f=w185) -> (s? t:f=w184:dbl)
    n273 = global write "Robot Global Data.vi" "Robot Angle"(w225) -> ()
    n274 = Less?(x=w194, y=w189) -> (x < y?=w235:bool)
    n275 = And(x=w171, y=w219) -> (x .and. y?=w211:bool)
    n276 = And(x=w171, y=w214) -> (x .and. y?=w212:bool)
    n277 = Not(x=w212) -> (.not. x?=w198:bool)
    n278 = Not(x=w211) -> (.not. x?=w199:bool)
    n279 = Select(t=w234, s=w235, f=w233) -> (s? t:f=w228:T28)
    n280 = call <vilib>:"WPI_EncoderGet.vi"("EncoderDevRef"=w207) -> ("Distance"=w204:dbl, "Rate"=w158:dbl)  [unwired: 5 in, 4 out]
    n281 = And(x=w199, y=w198) -> (x .and. y?=w210:bool)
    n282 = call <vilib>:"WPI_EncoderGet.vi"("EncoderDevRef"=w206) -> ("Distance"=w202:dbl, "Rate"=w161:dbl)  [unwired: 5 in, 4 out]
    n283 = Negate(x=w158) -> (-x=w157:dbl)
    n284 = Negate(x=w202) -> (-x=w180:dbl)
    "Drive Right" <- w180
    n285 = Negate(x=w161) -> (-x=w160:dbl)
    n286 = global write "Robot Global Data.vi" "Drive Right"(w180) -> ()
    n287 = Negate(x=w204) -> (-x=w203:dbl)
    n288 = Divide(x=w180, y=229.0) -> (x/y=→"Drive Right feet":dbl)
    n289 = Divide(x=w160, y="RateDivision") -> (x/y=w159:dbl)
    n290 = Negate(x=w203) -> (-x=w182:dbl)
    "Drive Left" <- w182
    n291 = global write "Robot Global Data.vi" "Drive Left Rate"(w159) -> ()
    n292 = Divide(x=w157, y="RateDivision") -> (x/y=w156:dbl)
    n293 = global write "Robot Global Data.vi" "Drive Right Rate"(w156) -> ()
    n294 = case shown="True" w211 {
      tunnel: w209 -> [_ w361]
      tunnel: w179 -> [_ w372]
      frame False {
        n295 = global read "Robot Global Data.vi" "ArcadeEnabled"() -> (w354:bool)
        n296 = case shown="False" w354 {
          frame False {
            n297 = global write "Robot Global Data.vi" "AutoDriveL"(0.0 ("Xaxis Addition")) -> ()
          }
          frame True {
          }
        }
      }
      frame True {
        # ".9"
        n298 = global write "Robot Global Data.vi" "ArcadeEnabled"(FALSE ("ArcadeEnabled")) -> ()
        n299 = call-poly <vilib>:"PID.vi"("output range"=cluster{"output high":dbl, "output low":dbl} {"output high"=0.6, "output low"=-0.6} ("Encoder Range"), "PID gains"="Encoder PID gains", "process variable"=w372, "setpoint"=w361) -> ("output"=w362:dbl)  [unwired: 6 in, 1 out]
        n300 = Greater?(x=w362, y=0.0) -> (0:w368:bool)
        n301 = Select(t=0.9, s=w368, f=-0.2) -> (s? t:f=w364:dbl)
        n302 = Select(t=0.2, s=w368, f=-0.9 ("t")) -> (s? t:f=w365:dbl)
        n303 = In Range and Coerce(upper limit=w364, x=w362, lower limit=w365) -> (coerced(x)=w363:dbl)  [unwired: 1 out]
        n304 = Negate(x=w363) -> (-x=w358:dbl)
        n305 = Sign(1:w358) -> (0:w359:dbl)
        n306 = case shown="1" w359 {
          tunnel: w358 -> [w377 w378]
          tunnel: [w376 w379] -> w357
          frame -1, Default {
            n307 = Multiply(x=w377, y=1.0 ("Left Forward Mult")) -> (x*y=w376:dbl)
          }
          frame 1 {
            n308 = Multiply(x=w378, y=0.93 ("Left Back Mult")) -> (x*y=w379:dbl)
          }
        }
        n309 = Negate(x=w357) -> (-x=w356:dbl)
        n310 = global write "Robot Global Data.vi" "AutoDriveL"(w356) -> ()
      }
    }
    n311 = case shown="True" w212 {
      tunnel: w209 -> [_ w335]
      tunnel: w178 -> [_ w334]
      frame False {
        n312 = global read "Robot Global Data.vi" "ArcadeEnabled"() -> (w327:bool)
        n313 = case shown="False" w327 {
          frame False {
            n314 = global write "Robot Global Data.vi" "AutoDriveR"(0.0 ("Xaxis Addition")) -> ()
          }
          frame True {
          }
        }
      }
      frame True {
        # ".9"
        n315 = global write "Robot Global Data.vi" "ArcadeEnabled"(FALSE ("ArcadeEnabled")) -> ()
        n316 = call-poly <vilib>:"PID.vi"("output range"=cluster{"output high":dbl, "output low":dbl} {"output high"=0.6, "output low"=-0.6} ("Encoder Range"), "PID gains"="Encoder PID gains 2", "process variable"=w334, "setpoint"=w335) -> ("output"=w336:dbl)  [unwired: 6 in, 1 out]
        n317 = Greater?(x=w336, y=0.0) -> (0:w341:bool)
        n318 = Select(t=0.9, s=w341, f=-0.2) -> (s? t:f=w337:dbl)
        n319 = Select(t=0.2, s=w341, f=-0.9 ("t")) -> (s? t:f=w338:dbl)
        n320 = In Range and Coerce(upper limit=w337, x=w336, lower limit=w338) -> (coerced(x)=w347:dbl)  [unwired: 1 out]
        n321 = Negate(x=w347) -> (-x=w332:dbl)
        n322 = Sign(1:w332) -> (0:w333:dbl)
        n323 = case shown="-1, Default" w333 {
          tunnel: w332 -> [w350 w351]
          tunnel: [w349 w352] -> w330
          frame -1, Default {
            n324 = Multiply(x=w350, y=0.93 ("Right Forward Mult")) -> (x*y=w349:dbl)
          }
          frame 1 {
            n325 = Multiply(x=w351, y=1.0 ("Right Back Mult")) -> (x*y=w352:dbl)
          }
        }
        n326 = Negate(x=w330) -> (-x=w329:dbl)
        n327 = global write "Robot Global Data.vi" "AutoDriveR"(w329) -> ()
      }
    }
    n328 = case shown="True" w210 {
      frame False {
      }
      frame True {
        n329 = global write "Robot Global Data.vi" "ArcadeEnabled"(TRUE ("ArcadeEnabled")) -> ()
      }
    }
    n330 = call <vilib>:"WPI_MotorControlSetOutput.vi"("Output"=w144, "MotorControlDevRef"=w249) -> ()  [unwired: 7 in, 3 out]
    n331 = global write "Robot Global Data.vi" "Drive Left"(w182) -> ()
    n332 = Divide(x=w182, y=226.58) -> (x/y=→"Drive Left feet":dbl)
    n333 = Unbundle By Name(w228) -> ("Center Position"=w229:cluster{"X":dbl, "Y":dbl})
    n334 = Unbundle By Name(w229) -> ("Y"=w227:dbl)
    n335 = Less?(x=w227, y=w184) -> (x < y?=w232:bool)
    n336 = Select(t=w228, s=w232, f=w231) -> (s? t:f=w230:T28)
    n337 = Unbundle By Name(w230) -> ("Center Position"=w242:cluster{"X":dbl, "Y":dbl}, "Distance (ft)"=w244:dbl)
    n338 = global write "Robot Global Data.vi" "Distance"(w244) -> ()
    n339 = Unbundle By Name(w242) -> ("X"=w243:dbl)
    n340 = global write "Robot Global Data.vi" "Center"(w243) -> ()
  }
  n341 = disable-structure shown="Disabled" {
    frame Disabled {
      n342 = disable-structure shown="Enabled" {
        disable-tunnel: [w508 1.0 ("SetFeeder")] -> w505
        frame Disabled {
          n343 = global read "Robot Global Data.vi" "DSFeederS"() -> (w511:dbl)
          n344 = Multiply(x=w511, y=-0.142 ("Xaxis Addition")) -> (x*y=w509:dbl)
          n345 = Add(x=0.68 ("Xaxis Addition"), y=w509) -> (x+y=w508:dbl)
        }
        frame Enabled {
        }
      }
      n346 = global write "Robot Global Data.vi" "Xaxis Addition"(0.0 ("Xaxis Addition")) -> ()
      n347 = global write "Robot Global Data.vi" "Line Up State"(enum16{"Default", "Gyro"}."Default" ("Line Up State")) -> ()
      n348 = global write "Robot Global Data.vi" "SetFeeder"(w505) -> ()
      n349 = global write "Robot Global Data.vi" "Encoder PID"(FALSE ("Encoder PID")) -> ()
    }
    frame Enabled {
    }
  }
